vi "QNET_Rotpen_Construct_State_Sim - Dera.vi"(2 "alpha (rad)":dbl, 3 "theta (rad)":dbl, 4 "alpha_r (rad)":dbl, 5 "theta_r (rad)":dbl) -> (0 "x cluster":T1, 1 "x array":dbl[](array[numeric]))   [LabVIEW 2021]
uses:
  <vilib>/Simulation/Implementation/Shared/SIMSCR Execution Mode.ctl
  <vilib>/Simulation/Scripting/Companion Diagram/SimConfigNode/SimParams.ctl
  <vilib>/Simulation/Scripting/Companion Diagram/SimConfigNode/_simSolvers.ctl
  <vilib>/Simulation/Param Hierarchy/Typedefs/SIMPH Param Control Actions.ctl
  <vilib>/Simulation/Implementation/Shared/NILVSim_ParamChanged.vi
  <vilib>/Simulation/Implementation/Shared/NILVSIM_BeginStep.vi
  <vilib>/Simulation/ContinuousLinear/Implementation/NILVSim Transfer Function Direct.llb/SIM Transfer Function Direct (SISO).vi
  <vilib>/Simulation/Implementation/Shared/NILVSim_Manager.vi
  <vilib>/Utility/error.llb/Clear Errors.vi
  <vilib>/Simulation/Implementation/Shared/NILVSim_FinalizeModel.vi
  <vilib>/Simulation/Implementation/Shared/SIM Unbundle Sim Info.vi
  <vilib>/Simulation/Implementation/Shared/SIMSH Read Queue.vi
  <vilib>/Simulation/Implementation/Shared/NILVSim_Initialize.vi
  <vilib>/Simulation/Utility/Implementation/NILVSim Get Time and IsAcceptedStep.vi
  <vilib>/Simulation/Implementation/Shared/NILVSim_GetModelError.vi
  <vilib>/Simulation/Implementation/Shared/SIM SimErrorHandler.vi
  <vilib>/Simulation/Implementation/Shared/SIM Bundle Sim Info.vi
  <vilib>/Simulation/Scripting/Companion Diagram/SimConfigNode/SimDog.xnode
  <vilib>/Simulation/Implementation/XNodeFramework/SimXNode/SimX.xnode
  <vilib>/Simulation/Implementation/Shared/NI_SIM_Implementation.lvlib
panel:
  in  "x":T1
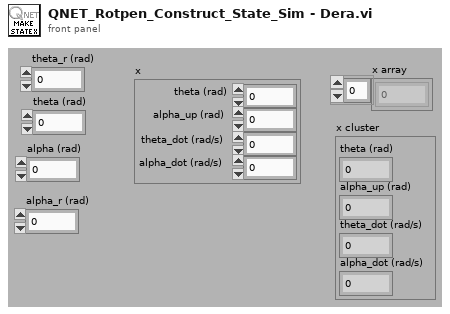
[diagram p1: front panel]
types:
  T1 = cluster{"theta (rad)":dbl, "alpha_up (rad)":dbl, "theta_dot (rad/s)":dbl, "alpha_dot (rad/s)":dbl}
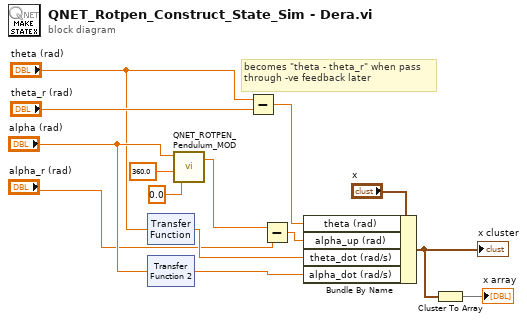
[diagram p0: block diagram]
diagram:
  # "becomes \"theta - theta_r\" when pass through -ve feedback later"
  n1 = xnode ("Transfer Function")("input u(t)"="theta (rad)") -> ("output y(t)"=w7:dbl)  [unwired: 4 in, 1 out]
  n2 = xnode ("Transfer Function 2")("input u(t)"="alpha (rad)") -> ("output y(t)"=w8:dbl)  [unwired: 4 in, 1 out]
  n3 = call "QNET_ROTPEN_Pendulum_MOD.vi"("offset (deg)"=0.0, "mod angle (deg)"=360.0, "gamma (rad)"="alpha (rad)") -> ("gamma mod (rad)"=w12:dbl)  [unwired: 1 in, 1 out]
  n4 = Subtract ("Subtract 2")(x="theta (rad)", y="theta_r (rad)") -> (x-y=w2:dbl)
  n5 = Subtract(x=w12, y="alpha_r (rad)") -> (x-y=w14:dbl)
  n6 = Bundle By Name(cluster="x", "theta (rad)"=w2, "alpha_up (rad)"=w14, "theta_dot (rad/s)"=w7, "alpha_dot (rad/s)"=w8) -> (w5:T1)
  "x cluster" <- w5
  n7 = Cluster To Array(cluster=w5) -> (array=→"x array":dbl[])
